vi "Close Log File.vi"(8 "error in (no error)":errorcluster, 11 "file refnum":refnum<file>) -> (0 "error out":errorcluster)   [LabVIEW 2021, in "DSF Core.lvlib" / "Logging Thread.lvclass"]
uses:
  Logging Thread.lvclass
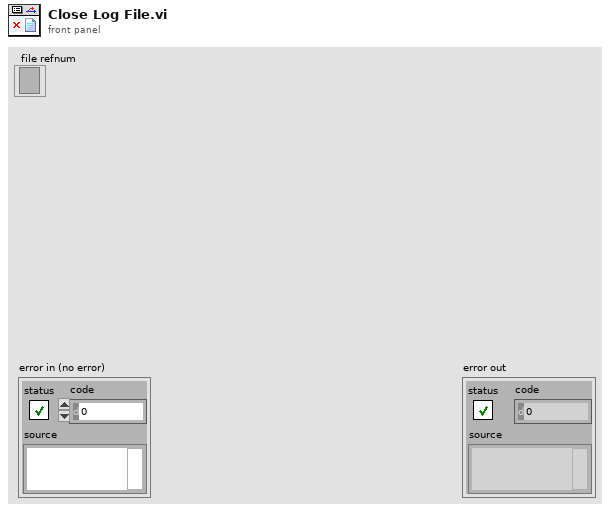
[diagram p1: front panel]
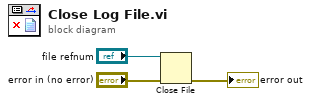
[diagram p0: block diagram]
diagram:
  n1 = Close File(refnum="file refnum", error in="error in (no error)") -> (error out=→"error out":errorcluster)  [unwired: 1 out]
